vi "half data samping.vi"() -> ()   [LabVIEW 2015]
panel:
  out "배열":string[](array[string])
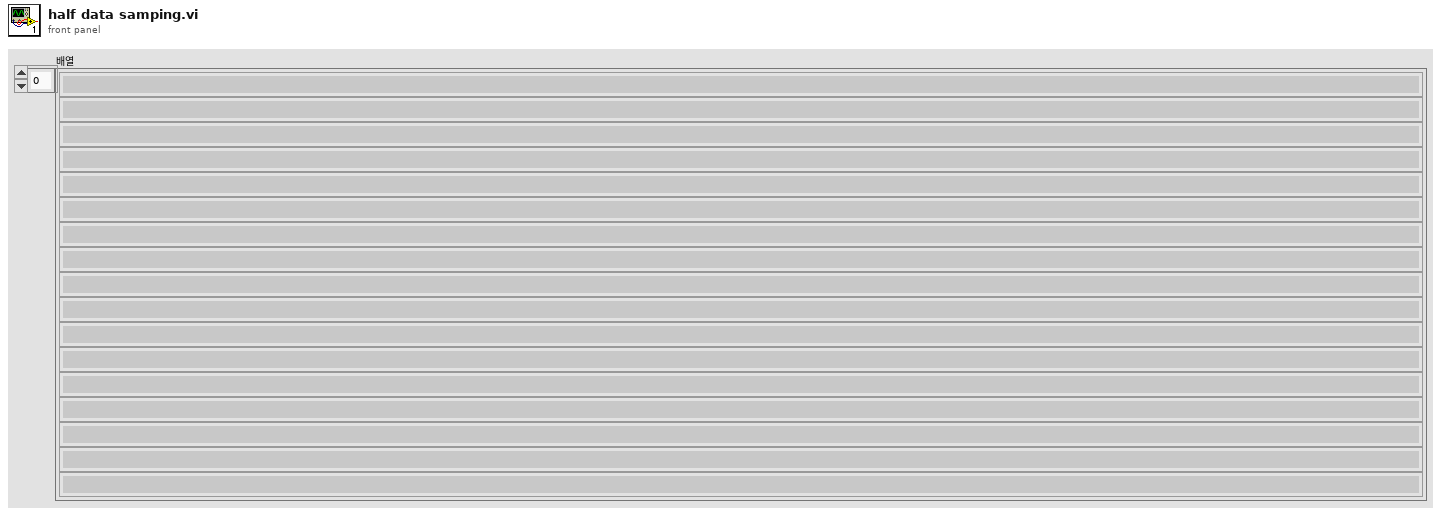
[diagram p1: front panel]
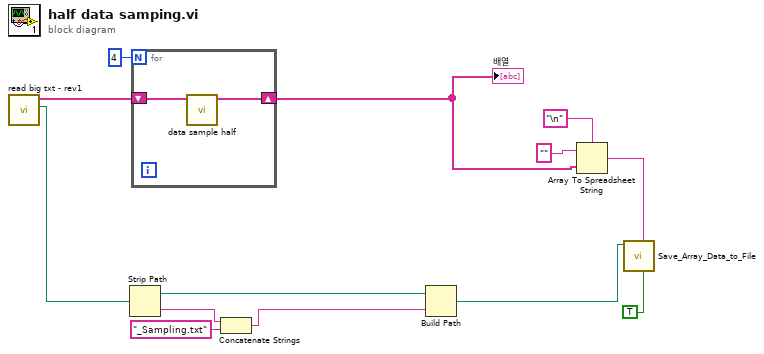
[diagram p0: block diagram]
diagram:
  n1 = call "read big txt - rev1.vi"() -> ("selected path"=w4:path, "배열"=w5:string[])  [unwired: 10 in]
  n2 = Strip Path(path=w4) -> (stripped path=w10:path, name=w9:string)
  n3 = for {
    N: 4 -> [_]
    shift-right: [w15] -> w1
    shift-left: w5 -> [w14]
    n4 = call "data sample half.vi"("배열"=w14) -> ("배열 2"=w15:string[])  [unwired: 10 in]
  }
  "배열" <- w1
  n5 = Concatenate Strings(w9, "_Sampling.txt" ("문자열")) -> (w7:string)
  n6 = Build Path(base path=w10, name or relative path=w7) -> (appended path=w6:path)
  n7 = Array To Spreadsheet String(delimiter (Tab)="\n" ("구분 문자(탭)"), array=w1, 3:"" ("포맷 문자열")) -> (spreadsheet string=w2:string)
  n8 = call "Save_Array_Data_to_File.vi"("Raw Stiring?"=TRUE, "Raw String"=w2, "file path (use dialog)"=w6) -> ()  [unwired: 8 in, 1 out]
